vi "send_book.vi"(5 "client id":string, 7 "start time":u32, 8 "error in (no error)":errorcluster, 9 "book":string, 10 "title":string, 11 "client tcp ref":refnum<k5>) -> (0 "error out":errorcluster, 2 "log string":string, 3 "client tcp ref out":refnum<k5>)   [LabVIEW 2020, in "librarian.lvclass"]
uses:
  librarian.lvclass
  shared/message--cluster.ctl
  shared/request--enum.ctl
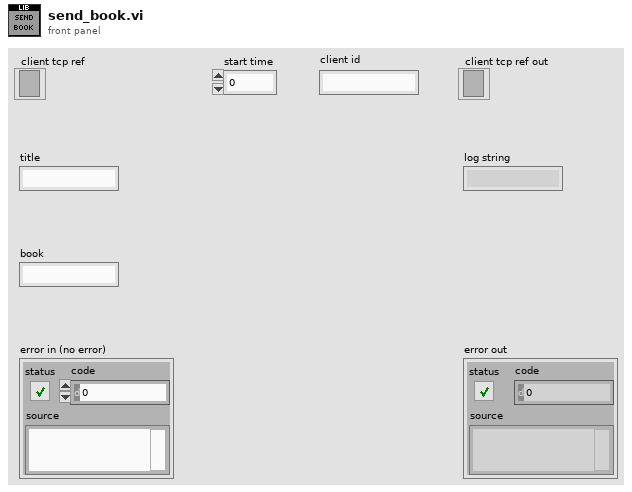
[diagram p1: front panel]
types:
  T1 = typedef "request--enum.ctl" = enum16{"CHECKIN", "CHECKOUT"}
  T2 = typedef "message--cluster.ctl" = cluster{"header":string, "cmd":T1, "title":string, "book":string}
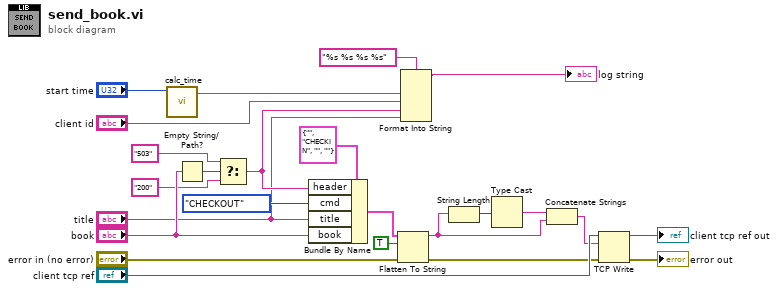
[diagram p0: block diagram]
diagram:
  n1 = call "calc_time.vi"("start time"="start time") -> ("String"=w9:string)  [unwired: 10 in]
  n2 = Empty String/Path?(string/path="book") -> (empty?=w14:bool)
  n3 = Select(t="503" ("header"), s=w14, f="200" ("header")) -> (s? t:f=w7:string)
  n4 = Bundle By Name(cluster=T2 {"header"="", "cmd"=enum."CHECKIN", "title"="", "book"=""} ("request"), "header"=w7, "cmd"=request--enum."CHECKOUT", "title"="title", "book"="book") -> (w22:T2)
  n5 = Flatten To String(anything=w22, prepend array or string size? (T)=TRUE, error in (no error)="error in (no error)") -> (data string=w2:string, error out=w18:errorcluster)  [unwired: 1 in, 1 out]
  n6 = Format Into String(format string="%s %s %s %s", w9, "client id", w7, "title") -> (resulting string=→"log string":string)  [unwired: 2 in, 1 out]
  n7 = String Length(string=w2) -> (length=w4:i32)
  n8 = Type Cast(x=w4) -> (*(type *) &x=w3:string)  [unwired: 1 in]
  n9 = Concatenate Strings(w3, w2) -> (w1:string)
  n10 = TCP Write(connection ID="client tcp ref", data in=w1, error in (no error)=w18) -> (connection ID out=→"client tcp ref out":refnum<k5>, error out=→"error out":errorcluster)  [unwired: 2 out]
